vi "Type.vi"(11 "BooleanPanel in":refnum<class "BooleanPanel.lvclass">) -> (2 "Type":refnum<class "Type.lvclass">)   [LabVIEW 2020, in "Conditum-Tools.lvlib" / "BooleanPanel.lvclass"]
uses:
  BooleanPanel.lvclass
  Conditum-Clone/Columns/Type/Type.lvclass
  Conditum-Clone/Columns/Boolean/Boolean.lvclass
  C:/dev/lv20CE/lv-conditum-tools/Conditum-Clone/Columns/Type/Type.lvclass
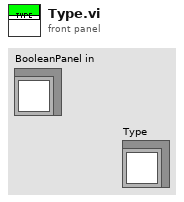
[diagram p1: front panel]
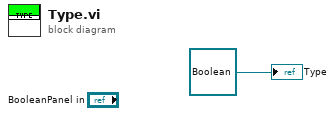
[diagram p0: block diagram]
diagram:
  "Type" <- refnum<class "Boolean.lvclass"> refnum ("Conditum:Columns:Boolean.lvclass")
